vi "DAQ_SV Gen Configure and Generate.vi"(0 "DAQmx Task In":refnum<k21>, 5 "Range and Terminal Settings":T1={"Min Voltage (V)"=-10.0, "Max Voltage (V)"=10.0} {"Max Voltage (V)" format="%.2p"; "Min Voltage (V)" format="%.2p"}, 7 "Signal Generation Settings":T2={"Generation Type"=enum."Single Tone", "Generation Time (s)"=0.1, "Voltage Offset (v)"=0.0, "Single Tone Settings"={"Waveform Type"=enum."Sine Wave", "Frequency (Hz)"=100.0, "Amplitude (V)"=1.0, "Duty Cycle (%)"=50.0}, "Multi Tone Settings"=[]} {"Voltage Offset (v)" format="%.2p"; "Generation Time (s)" format="%.2p"; "Multi Tone Settings"."Amplitude (V)" format="%.2p"; "Multi Tone Settings"."Frequency (Hz)" format="%.2p"; "Single Tone Settings"."Duty Cycle (%)" format="%.2p"; "Single Tone Settings"."Amplitude (V)" format="%.2p"; "Single Tone Settings"."Frequency (Hz)" format="%.2p"}, 9 "Timing & Trigger Settings":T7={"Trigger Settings"={"Trigger Type"=enum."No Trigger", "Digital Start Trigger Source"="", "Digital Start Trigger Edge"=10280}, "Timing Settings"={"Sample Clock Source"="OnboardClock", "Sample Rate (Hz)"=100000.0}} {"Timing Settings"."Sample Rate (Hz)" format="%.2p"; "Trigger Settings"."Digital Start Trigger Edge" items=["Rising"=10280, "Falling"=10171]}, 11 "error in":errorcluster) -> (4 "DAQmx Task Out":refnum<k21>, 6 "Generated Voltage Waveforms":waveform(dbl)[](graph), 15 "error out":errorcluster)   [LabVIEW 2021, in "DAQ_Signal Voltage Generation.lvlib"]
doc: "Configure, initiate and generate signal voltage waveforms from the channels configured."
uses:
  DAQ_Signal Voltage Generation.lvlib
  Typedefs/Range and Terminal Settings.ctl
  Typedefs/Signal Generation Settings.ctl
  Typedefs/Generation Types.ctl
  Typedefs/Single Tone Settings.ctl
  Typedefs/Waveform Type.ctl
  Typedefs/Tone Settings.ctl
  Typedefs/Timing & Trigger Settings.ctl
  Typedefs/Trigger Settings.ctl
  Typedefs/Timing Settings.ctl
  <vilib>/DAQmx/write.llb/DAQmx Write (Analog 1D Wfm NChan NSamp).vi
  <vilib>/DAQmx/configure/timing.llb/DAQmx Timing (Sample Clock).vi
  <vilib>/DAQmx/configure/trigger.llb/DAQmx Start Trigger (Digital Edge).vi
  <vilib>/DAQmx/miscellaneous.llb/DAQmx Fill In Error Info.vi
  <resource>/objmgr/daqmx.rc
panel:
  # "Outputs"
  # "Inputs"
  # "Frequency (Hz)"
  # "Amplitude (V)"
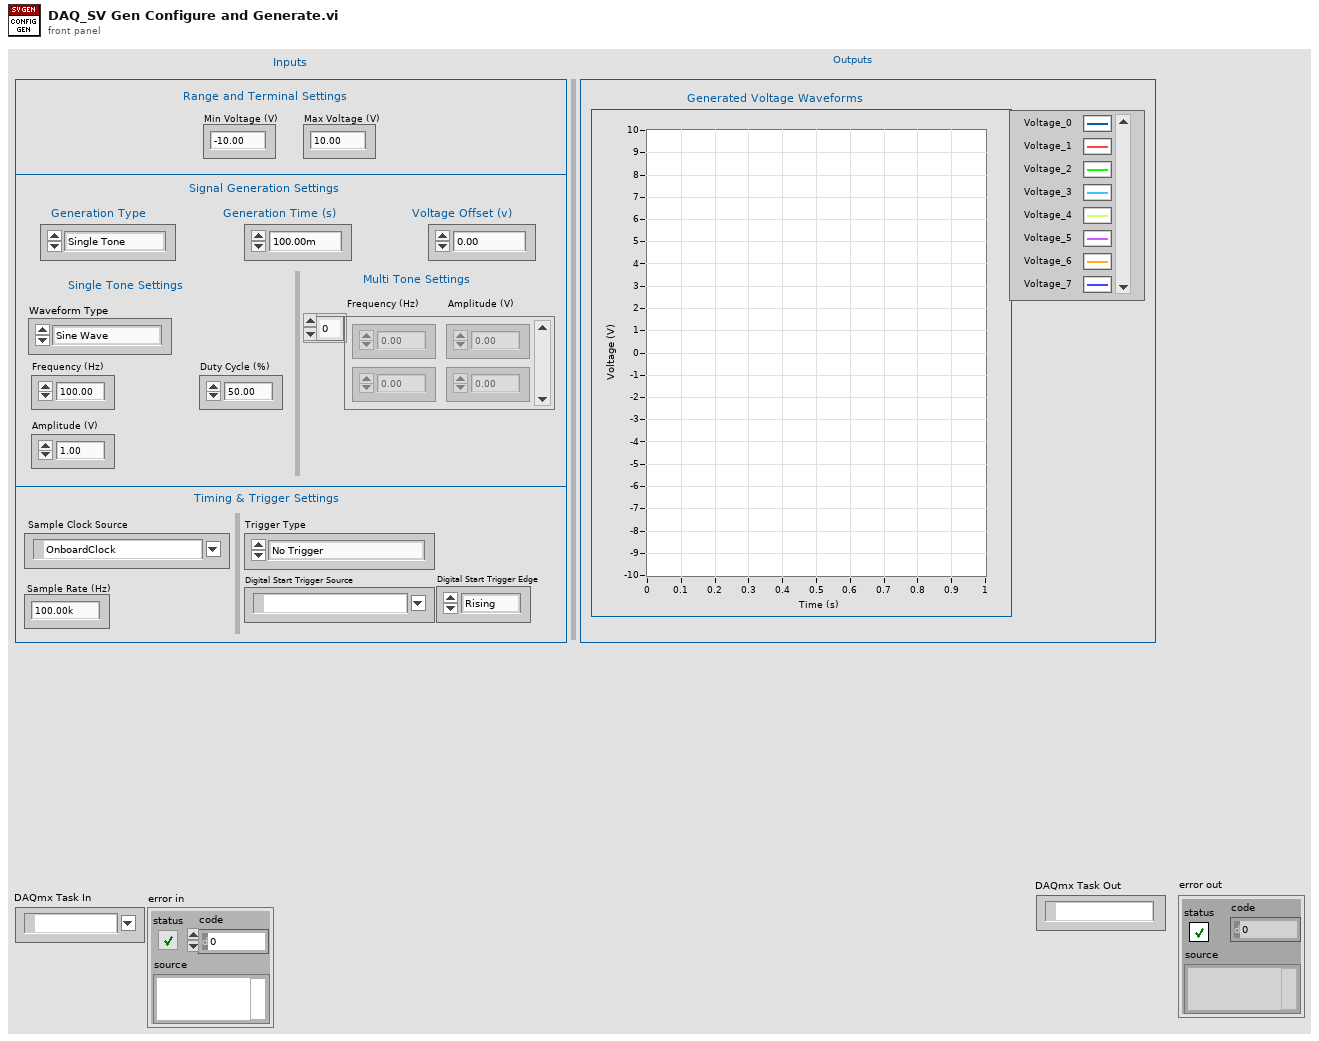
[diagram p1: front panel]
types:
  T1 = typedef "DAQ_Signal Voltage Generation.lvlib/Range and Terminal Settings.ctl" = cluster{"Min Voltage (V)":dbl, "Max Voltage (V)":dbl}
  T2 = typedef "DAQ_Signal Voltage Generation.lvlib/Signal Generation Settings.ctl" = cluster{"Generation Type":T3, "Generation Time (s)":dbl, "Voltage Offset (v)":dbl, "Single Tone Settings":T4, "Multi Tone Settings":T6[]}
  T3 = typedef "DAQ_Signal Voltage Generation.lvlib/Generation Types.ctl" = enum16{"Single Tone", "Multi Tone"}
  T4 = typedef "DAQ_Signal Voltage Generation.lvlib/Single Tone Settings.ctl" = cluster{"Waveform Type":T5, "Frequency (Hz)":dbl, "Amplitude (V)":dbl, "Duty Cycle (%)":dbl}
  T5 = typedef "DAQ_Signal Voltage Generation.lvlib/Waveform Type.ctl" = enum16{"Sine Wave", "Square Wave"}
  T6 = typedef "DAQ_Signal Voltage Generation.lvlib/Tone Settings.ctl" = cluster{"Frequency (Hz)":dbl, "Amplitude (V)":dbl}
  T7 = typedef "DAQ_Signal Voltage Generation.lvlib/Timing & Trigger Settings.ctl" = cluster{"Trigger Settings":T8, "Timing Settings":T9}
  T8 = typedef "DAQ_Signal Voltage Generation.lvlib/Trigger Settings.ctl" = cluster{"Trigger Type":enum16{"No Trigger", "Digital Start"}, "Digital Start Trigger Source":tag, "Digital Start Trigger Edge":i32}
  T9 = typedef "DAQ_Signal Voltage Generation.lvlib/Timing Settings.ctl" = cluster{"Sample Clock Source":tag, "Sample Rate (Hz)":dbl}
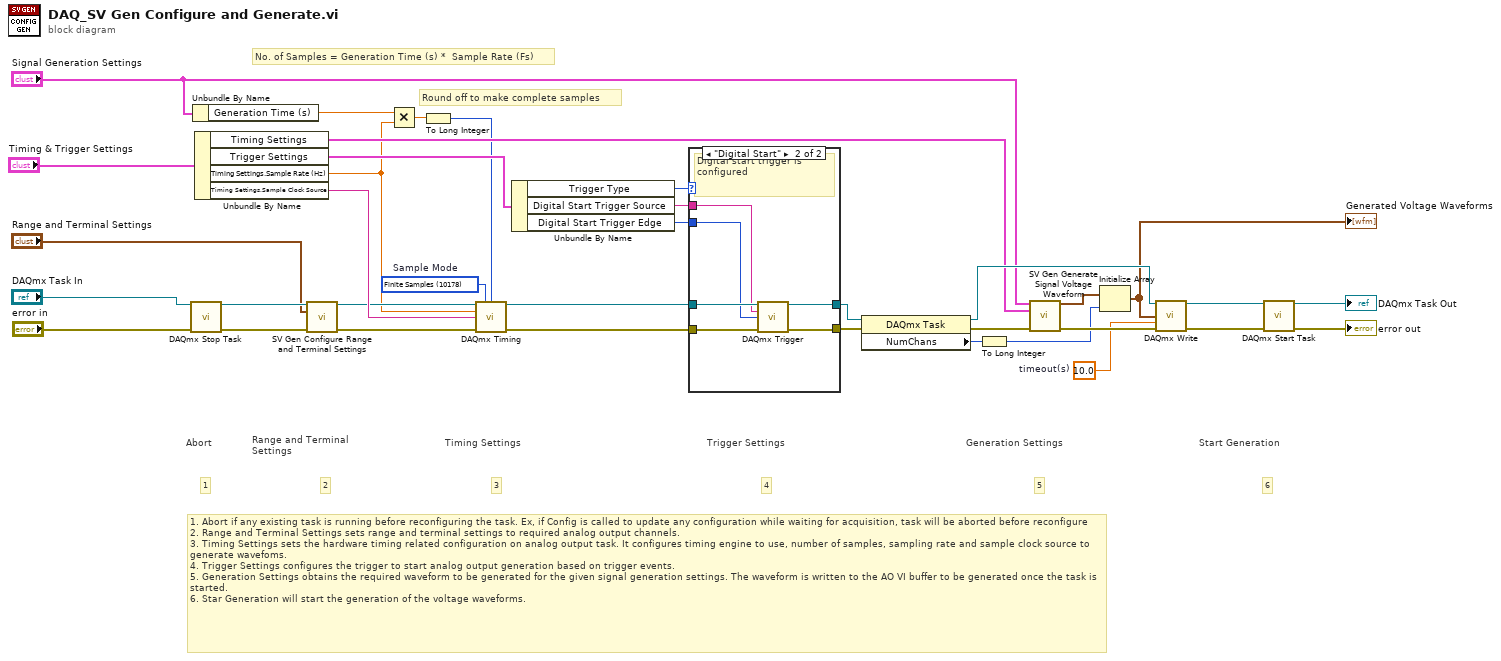
[diagram p0: block diagram]
diagram:
  w1 = 10.0  # timeout(s)
  w30 = 10178 items=["Finite Samples"=10178, "Continuous Samples"=10123, "Hardware Timed Single Point"=12522]  # Sample Mode
  # "6"
  # "1"
  # "Abort"
  # "Round off to make complete samples"
  # "No. of Samples = Generation Time (s) *  Sample Rate (Fs)"
  # "5"
  # "Start Generation"
  # "4"
  # "Generation Settings"
  # "3"
  # "2"
  # "Range and Terminal \nSettings"
  # "Trigger Settings"
  # "Timing Settings"
  # "1. Abort if any existing task is running before reconfiguring the task. Ex, if Config is called to update any configuration while waiting for acquisition, task will be aborted before reconfigure\n2. Range and Terminal Settings sets range and terminal settings to required analog output channels.\n3. Timing Settings sets the hardware timing related configuration on analog output task. It configures timing engine to use, number of samples, sampling rate and sample clock source to generate wavefoms.\n4. Trigger Settings configures the trigger to start analog output generation based on trigger events.\n5. Generation Settings obtains the required waveform to be generated for the given signal generation settings. The waveform is written to the AO VI buffer to be generated once the task is started.\n6. Star Generation will start the generation of the voltage waveforms."
  n1 = call <vilib>:"DAQmx Stop Task.vi"("task/channels in"="DAQmx Task In", "error in"="error in") -> ("task out"=w22:refnum<k21>, "error out"=w21:errorcluster)  [unwired: 12 in]
  n2 = Unbundle By Name("Signal Generation Settings") -> ("Generation Time (s)"=w5:dbl)
  n3 = Unbundle By Name("Timing & Trigger Settings") -> ("Timing Settings"=w8:T9, "Trigger Settings"=w23:T8, "Timing Settings.Sample Rate (Hz)"=w4:dbl, "Timing Settings.Sample Clock Source"=w29:tag)
  n4 = call "SV Gen Configure Range and Terminal Settings.vi"("DAQmx Task In"=w22, "Range and Terminal Settings"="Range and Terminal Settings", "error in (no error)"=w21) -> ("DAQmx Task Out"=w24:refnum<k21>, "error out"=w25:errorcluster)  [unwired: 11 in]
  n5 = Multiply(x=w5, y=w4) -> (x*y=w3:dbl)
  n6 = To Long Integer(number=w3) -> (32bit integer=w2:i32)
  n7 = call-poly <vilib>:"DAQmx Timing.vi"("task/channels in"=w24, "sample mode"=w30, "samples per channel"=w2, "rate"=w4, "source"=w29, "error in"=w25) -> ("task out"=w20:refnum<k21>, "error out"=w19:errorcluster)  [unwired: 8 in]
  n8 = Unbundle By Name(w23) -> ("Trigger Type"=w26:enum16{"No Trigger", "Digital Start"}, "Digital Start Trigger Source"=w28:tag, "Digital Start Trigger Edge"=w27:i32)
  n9 = case shown="\"Digital Start\"" w26 {
    tunnel: w20 -> [w38 w44]
    tunnel: w19 -> [w37 w43]
    tunnel: [w38 w42] -> w15
    tunnel: [w37 w41] -> w16
    tunnel: w28 -> [_ w40]
    tunnel: w27 -> [_ w39]
    frame Default {
      # "No Trigger settings has been configured"
    }
    frame "Digital Start" {
      # "Digital start trigger is configured"
      n10 = call-poly <vilib>:"DAQmx Trigger.vi"("task/channels in"=w44, "source"=w40, "edge"=w39, "error in"=w43) -> ("task out"=w42:refnum<k21>, "error out"=w41:errorcluster)  [unwired: 10 in]
    }
  }
  n11 = property class="DAQmx Task"(reference=w15, error in=w16) -> (reference out=w14:refnum<k21>, error out=w11:errorcluster, "NumChans"=w13:u32)
  n12 = To Long Integer(number=w13) -> (32bit integer=w12:i32)
  n13 = call "SV Gen Generate Signal Voltage Waveform.vi"("Signal Generation Settings"="Signal Generation Settings", "Timing Settings"=w8, "error in"=w11) -> ("Generated Voltage Waveforms"=w17:waveform(dbl), "error out"=w18:errorcluster)  [unwired: 11 in]
  n14 = Initialize Array(w17, w12) -> (w10:waveform(dbl)[])
  "Generated Voltage Waveforms" <- w10
  n15 = call-poly <vilib>:"DAQmx Write.vi"("task/channels in"=w14, "data"=w10, "timeout"=w1, "error in"=w18) -> ("task out"=w35:refnum<k21>, "error out"=w36:errorcluster)  [unwired: 9 in, 1 out]
  n16 = call <vilib>:"DAQmx Start Task.vi"("task/channels in"=w35, "error in"=w36) -> ("task out"=→"DAQmx Task Out":refnum<k21>, "error out"=→"error out":errorcluster)  [unwired: 12 in]
